vi "TabPage_Vis.vi"(8 "error in":errorcluster, 9 "Visible? (F)":bool, 10 "Page (0)":i32, 11 "Tab_ref":refnum<vi>) -> (0 "error out":errorcluster)   [LabVIEW 2016]
doc: "Подпрограмма скрывает с лицевой панели\nвыбранную вкладку у принимаемого\n TAB Control Reference.\nНомер скрываемой вкладки и состояние\nтакже передается из основной программы"
panel:
  # "Подпрограмма скрывает с лицевой панели\nвыбранную вкладку у принимаемого\n TAB Control Reference.\nНомер скрываемой вкладки и состояние\nтакже передается из основной программы"
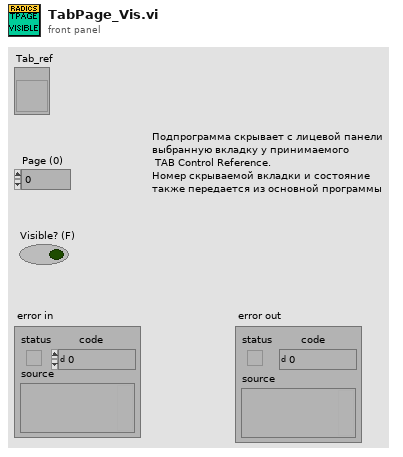
[diagram p1: front panel]
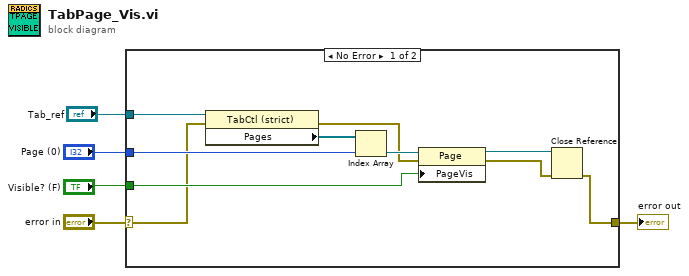
[diagram p0: block diagram]
diagram:
  n1 = case shown="No Error" "error in" {
    selector: "error in" -> [w8 w16]
    tunnel: [w7 w16] -> w4
    tunnel: "Page (0)" -> [w12 _]
    tunnel: "Visible? (F)" -> [w9 _]
    tunnel: "Tab_ref" -> [w6 _]
    frame No Error {
      n2 = property class="TabCtl (strict)"(reference=w6, error in=w8) -> (error out=w11:errorcluster, "Pages"=w13:refnum<vi>[])  [unwired: 1 out]
      n3 = Index Array(array=w13, index=w12) -> (element=w14:refnum<vi>)
      n4 = property class="Page"(reference=w14, error in=w11, "PageVis"=w9) -> (reference out=w15:refnum<vi>, error out=w10:errorcluster)
      n5 = Close Reference(reference=w15, error in (no error)=w10) -> (error out=w7:errorcluster)
    }
    frame Error {
    }
  }
  "error out" <- w4
